vi "PathPlanner_ReplanningConfig_GetAll.vi"() -> ()   [LabVIEW 2019, in "PathPlanner24.lvlib"]
doc: "Create a path replanning configuration\n\nInputs:\n@param enableInitialReplanning Should the path be replanned at the start of path following if\n * the robot is not already at the starting point?\n * @param enableDynamicReplanning Should the path be replanned if the error grows too large or if\n * a large error spike happens while following the path?\n * @param dynamicReplanningTotalErrorThreshold The total error threshold, in meters, that will\n * cause the path to be replanned\n * @param dynamicReplanningErrorSpikeThreshold The error spike threshold, in meters, that will\n * cause the path to be replanned\n\nOutputs:\n - ReplanningConfig - cluster - created data cluster"
uses:
  PathPlanner24.lvlib
  TypeDef/PathPlannerReplanningConfig.ctl
panel:
  out "dynamicReplanningErrorSpikeThreshold":dbl=0.25
  out "dynamicReplanningTotalErrorThreshold":dbl=1.0
  out "enableDynamicReplanning":bool
  out "enableInitialReplanning":bool=TRUE
  in  "ReplanningConfig":T1
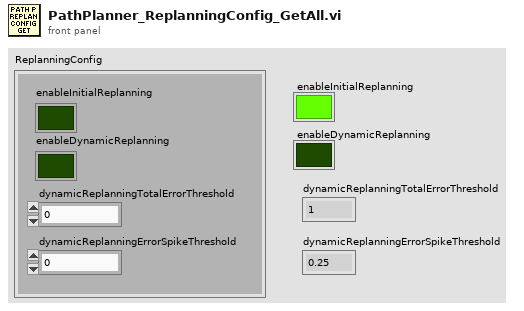
[diagram p1: front panel]
types:
  T1 = typedef "PathPlanner24.lvlib/PathPlannerReplanningConfig.ctl" = cluster{"enableInitialReplanning":bool, "enableDynamicReplanning":bool, "dynamicReplanningTotalErrorThreshold":dbl, "dynamicReplanningErrorSpikeThreshold":dbl}
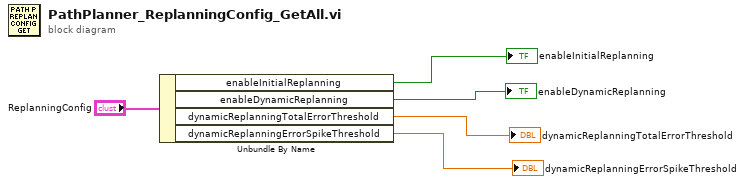
[diagram p0: block diagram]
diagram:
  n1 = Unbundle By Name("ReplanningConfig") -> ("enableInitialReplanning"=→"enableInitialReplanning":bool, "enableDynamicReplanning"=→"enableDynamicReplanning":bool, "dynamicReplanningTotalErrorThreshold"=→"dynamicReplanningTotalErrorThreshold":dbl, "dynamicReplanningErrorSpikeThreshold"=→"dynamicReplanningErrorSpikeThreshold":dbl)
